vi "LI-U8 compute 256 to power.vi"(4 "power (U32)":u32, 5 "X (U8)":u8) -> (1 "x* 256^Power":T1)   [LabVIEW 2013]
doc: "Returns in large number - U8 array format X * 256 to the input power."
uses:
  User Access Type defs/Large number - U8 array.ctl
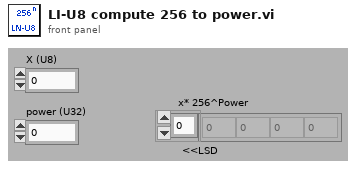
[diagram p1: front panel]
types:
  T1 = typedef "Large number - U8 array.ctl" = u8[]
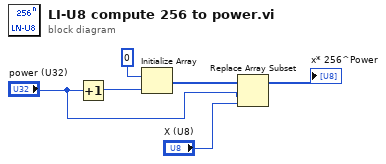
[diagram p0: block diagram]
diagram:
  n1 = Increment(x="power (U32)") -> (x+1=w5:u32)
  n2 = Initialize Array(u8 0 ("Numeric"), w5) -> (w4:u8[])
  n3 = Replace Array Subset(array=w4, new element="X (U8)", index="power (U32)") -> (→"x* 256^Power":u8[])
